vi "CheckIfClassAttrLocked.vi"(5 "error in (no error)":errorcluster) -> (15 "locked":bool, 19 "error out":errorcluster)   [LabVIEW 2020, in "G#BaseClass2.lvclass"]
uses:
  G#BaseClass2.lvclass
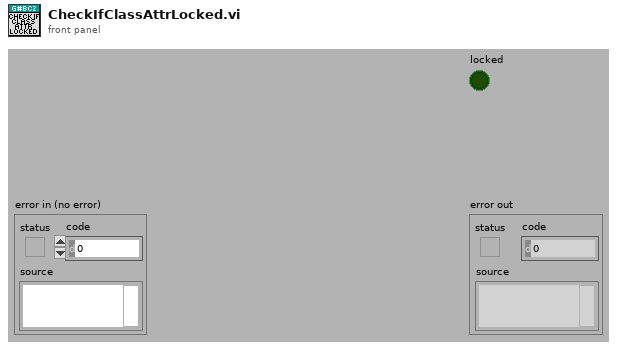
[diagram p1: front panel]
types:
  T1 = typedef "G#BaseClass2.lvclass/ClassAttributesRef.ctl" = refnum<data-value>
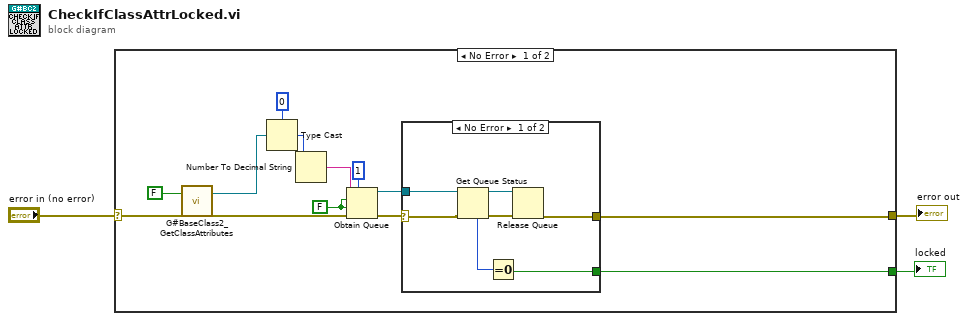
[diagram p0: block diagram]
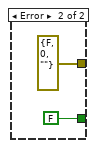
[diagram p2: hidden frame]
diagram:
  n1 = case shown="No Error" "error in (no error)" {
    selector: "error in (no error)" -> [w7 w26]
    tunnel: [w10 w26] -> w2
    tunnel: [w8 _] -> w1
    frame No Error {
      w15 = FALSE ("create if not found? (T)")
      n2 = call "G#BaseClass2_GetClassAttributes.vi"("return data? (T)"=FALSE ("return data"), "error in (no error)"=w7) -> ("class attributes ref"=w4:T1, "error out"=w6:errorcluster)  [unwired: 13 in, 3 out]
      n3 = Type Cast(type=u32 0, x=w4) -> (*(type *) &x=w12:u32)
      n4 = Number To Decimal String(number=w12) -> (decimal integer string=w16:string)  [unwired: 1 in]
      n5 = Obtain Queue(max queue size (-1, unlimited)=1, name (unnamed)=w16, element data type=w15, create if not found? (T)=w15, error in (no error)=w6) -> (queue out=w11:refnum<queue>, error out=w9:errorcluster)  [unwired: 1 out]
      n6 = case shown="No Error" w9 {
        selector: w9 -> [w19 _]
        tunnel: w11 -> [w23 _]
        tunnel: [w22 errorcluster {"status"=FALSE, "code"=0, "source"=""} ("error out")] -> w10
        tunnel: [w18 FALSE] -> w8
        frame No Error {
          n7 = Get Queue Status(queue=w23, error in (no error)=w19) -> (queue out=w20:refnum<queue>, error out=w21:errorcluster, # elements in queue=w17:i32)  [unwired: 1 in, 5 out]
          n8 = Equal To 0?(x=w17) -> (x = 0?=w18:bool)
          n9 = Release Queue(queue=w20, error in (no error)=w21) -> (error out=w22:errorcluster)  [unwired: 1 in, 2 out]
        }
        frame Error {
        }
      }
    }
    frame Error {
    }
  }
  "error out" <- w2
  "locked" <- w1
